vi "adam-ALL-IOs-panel.vi"(0 "VISA Refnum in":refnum<visa-resource-name>, 1 "ADAM-5000-data-current":T3, 3 "Digital Outputs":T4, 4 "Analog Outputs":T6, 5 "error in (no error)":errorcluster, 6 "Module Type":T10(ring), 7 "chassis-slot":i32=5, 9 "cmd-response in":T1, 10 "Chassis Settings":T8, 11 "reference":refnum<vi>) -> (12 "slot: x":T9, 14 "VISA Refnum out":refnum<visa-resource-name>, 15 "ADAM-5000-data-new":T3, 18 "cmd-response out":T1, 19 "error out":errorcluster)   [LabVIEW 2020]
uses:
  controls/digital-output-cluster.ctl
  controls/digitial-input-cluster.ctl
  controls/analog-input-cluster.ctl
  controls/thermocouple-input-cluster.ctl
  controls/adam-module-select-tab.ctl
  controls/adam-5000-serial-settings.ctl
  controls/analog-output-cluster.ctl
  controls/adam-5000-all-module-datas.ctl
  controls/adam-5000-cmd-response.ctl
panel:
  out "Analog Inputs":T2
  out "Digital Inputs":T5
  out "Thermocouple Inputs (degC)":T7
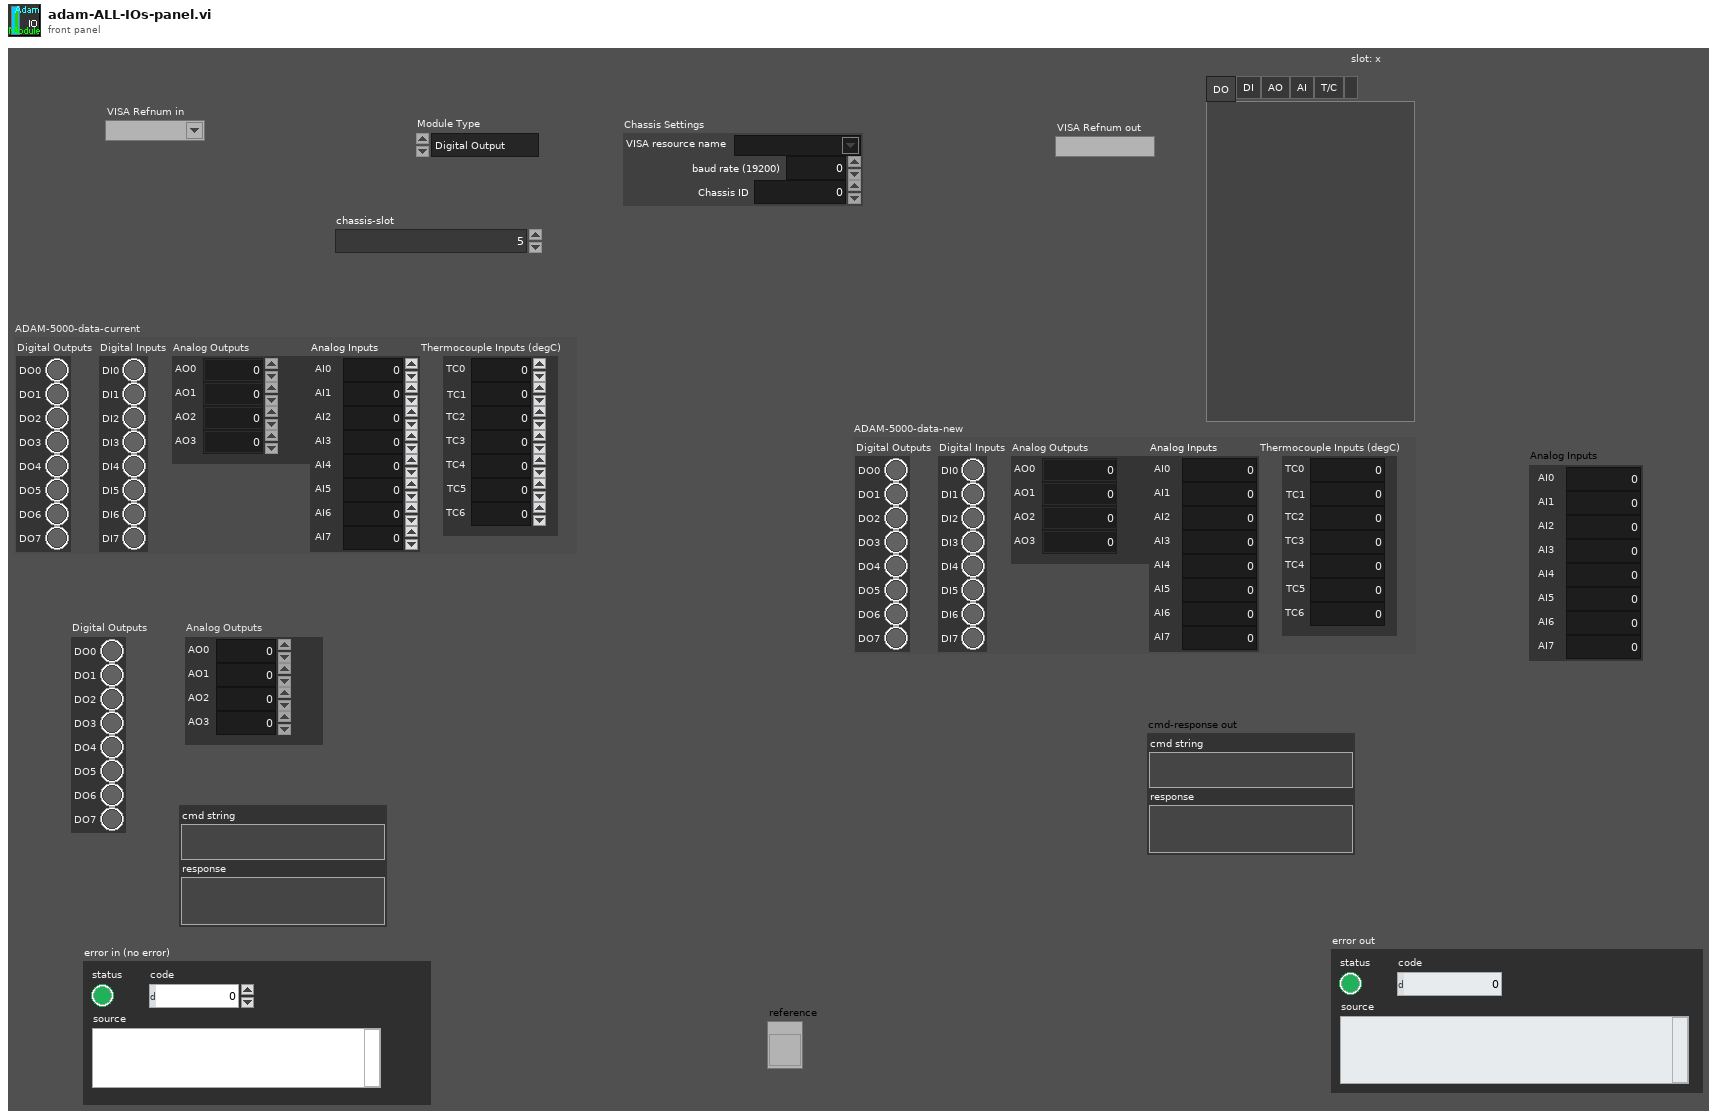
[diagram p1: front panel]
types:
  T1 = typedef "adam-5000-cmd-response.ctl" = cluster{"cmd string":string, "response":string}
  T2 = typedef "analog-input-cluster.ctl" = cluster{"AI0":dbl, "AI1":dbl, "AI2":dbl, "AI3":dbl, "AI4":dbl, "AI5":dbl, "AI6":dbl, "AI7":dbl}
  T3 = typedef "adam-5000-all-module-datas.ctl" = cluster{"Digital Outputs":T4, "Digital Inputs":T5, "Analog Outputs":T6, "Analog Inputs":T2, "Thermocouple Inputs (degC)":T7}
  T4 = typedef "digital-output-cluster.ctl" = cluster{"DO0":bool, "DO1":bool, "DO2":bool, "DO3":bool, "DO4":bool, "DO5":bool, "DO6":bool, "DO7":bool}
  T5 = typedef "digitial-input-cluster.ctl" = cluster{"DI0":bool, "DI1":bool, "DI2":bool, "DI3":bool, "DI4":bool, "DI5":bool, "DI6":bool, "DI7":bool}
  T6 = typedef "analog-output-cluster.ctl" = cluster{"AO0":dbl, "AO1":dbl, "AO2":dbl, "AO3":dbl}
  T7 = typedef "thermocouple-input-cluster.ctl" = cluster{"TC0":dbl, "TC1":dbl, "TC2":dbl, "TC3":dbl, "TC4":dbl, "TC5":dbl, "TC6":dbl}
  T8 = typedef "adam-5000-serial-settings.ctl" = cluster{"VISA resource name":refnum<visa-resource-name>, "baud rate (19200)":u32, "Chassis ID":u8}
  T9 = typedef "adam-module-select-tab.ctl" = enum32{"DO", "DI", "AO", "AI", "T/C", ""}
  T10 = enum16{"Digital Output", "Digital Input", "Analog Output", "Analog Input", "Thermocouple", "Power Relay", "empty"}
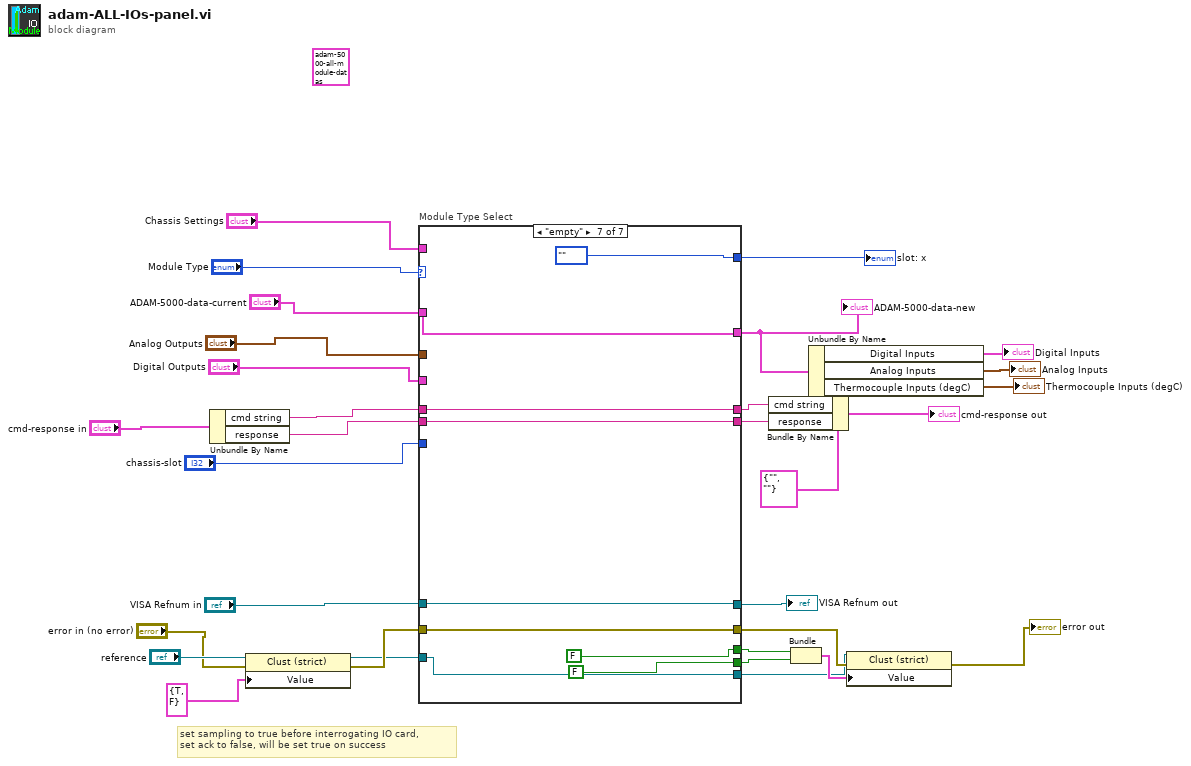
[diagram p0: block diagram]
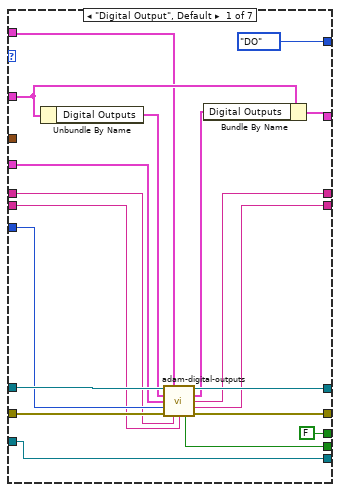
[diagram p2: hidden frame]
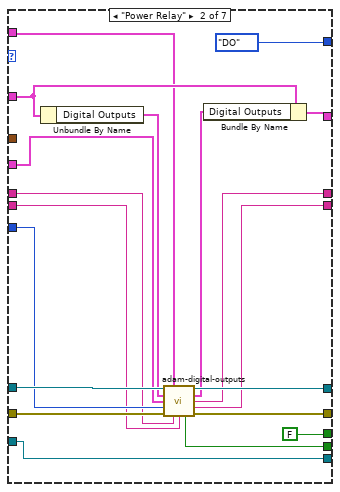
[diagram p3: hidden frame]
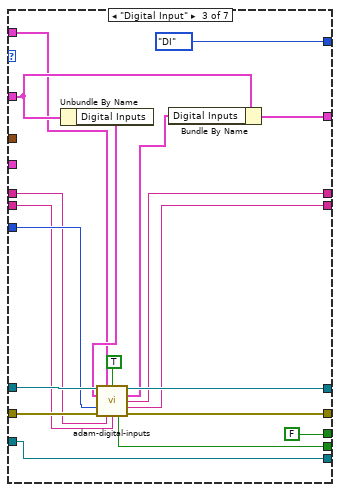
[diagram p4: hidden frame]
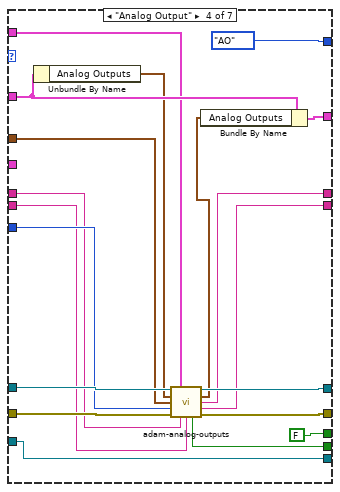
[diagram p5: hidden frame]
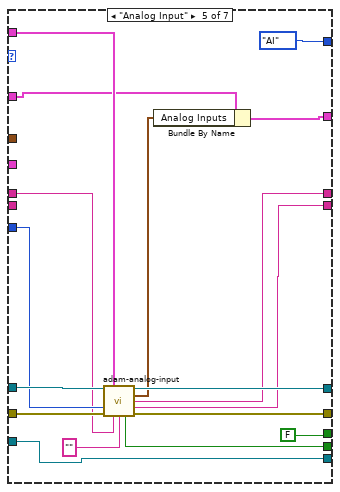
[diagram p6: hidden frame]
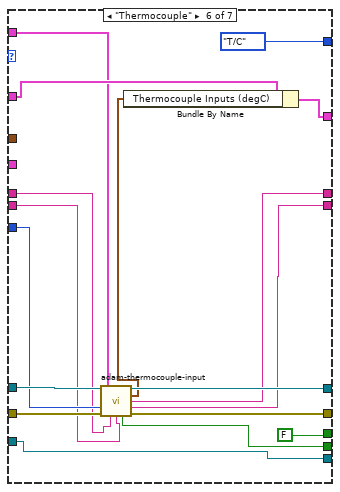
[diagram p7: hidden frame]
diagram:
  (unwired) T3 {"Digital Outputs"={"DO0"=FALSE, "DO1"=FALSE, "DO2"=FALSE, "DO3"=FALSE, "DO4"=FALSE, "DO5"=FALSE, "DO6"=FALSE, "DO7"=FALSE}, "Digital Inputs"={"DI0"=FALSE, "DI1"=FALSE, "DI2"=FALSE, "DI3"=FALSE, "DI4"=FALSE, "DI5"=FALSE, "DI6"=FALSE, "DI7"=FALSE}, "Analog Outputs"={"AO0"=0.0, "AO1"=0.0, "AO2"=0.0, "AO3"=0.0}, "Analog Inputs"={"AI0"=0.0, "AI1"=0.0, "AI2"=0.0, "AI3"=0.0, "AI4"=0.0, "AI5"=0.0, "AI6"=0.0, "AI7"=0.0}, "Thermocouple Inputs (degC)"={"TC0"=0.0, "TC1"=0.0, "TC2"=0.0, "TC3"=0.0, "TC4"=0.0, "TC5"=0.0, "TC6"=0.0}} ("ADAM-5000-data-typedefs")
  # "set sampling to true before interrogating IO card,\nset ack to false, will be set true on success"
  n1 = Unbundle By Name("cmd-response in") -> ("cmd string"=w19:string, "response"=w20:string)
  n2 = property on="Property Node" class="Clust (strict)"(reference="reference", error in="error in (no error)", "Value"=cluster{"Sampling":bool, "Ack":bool} {"Sampling"=TRUE, "Ack"=FALSE}) -> (reference out=w7:refnum<vi>, error out=w9:errorcluster)
  n3 = case "Module Type Select" shown="\"empty\"" "Module Type" {
    tunnel: "ADAM-5000-data-current" -> [w48 w67 w82 w106 w117 w141 w143]
    tunnel: [adam-module-select-tab."DO" ("slot: 0") adam-module-select-tab."DO" ("slot: 0") adam-module-select-tab."DI" ("slot: 0") adam-module-select-tab."AO" ("slot: 0") adam-module-select-tab."AI" ("slot: 0") adam-module-select-tab."T/C" ("slot: 0") adam-module-select-tab."" ("slot: 0")] -> w26
    tunnel: [w49 w68 w87 w105 w116 w140 w143] -> w24
    tunnel: "Chassis Settings" -> [w38 w57 w75 w97 w124 w134 _]
    tunnel: "chassis-slot" -> [w41 w60 w80 w98 w119 w133 _]
    tunnel: "VISA Refnum in" -> [w47 w66 w86 w102 w123 w138 w144]
    tunnel: w9 -> [w46 w65 w85 w104 w122 w137 w145]
    tunnel: [w45 w64 w84 w103 w121 w136 w145] -> w6
    tunnel: [w44 w63 w83 w101 w120 w135 w144] -> w28
    tunnel: [w39 w58 w76 w95 w118 w129 w147] -> w13
    tunnel: w20 -> [w36 w55 w78 w94 _ w131 w147]
    tunnel: w19 -> [w37 w56 w79 w93 w113 w132 w148]
    tunnel: [w34 w52 w71 w90 w109 w126 FALSE ("Sampling")] -> w17
    tunnel: [w40 w59 w77 w96 w114 w130 w148] -> w14
    tunnel: [FALSE ("cmd aknowledged") FALSE ("Sampling") FALSE ("Sampling") FALSE ("Sampling") FALSE ("Sampling") FALSE ("Sampling") FALSE ("cmd aknowledged")] -> w18
    tunnel: "Digital Outputs" -> [w35 w54 _ _ _ _ _]
    tunnel: "Analog Outputs" -> [_ _ _ w92 _ _ _]
    tunnel: w7 -> [w32 w51 w70 w89 w108 w125 w142]
    tunnel: [w32 w51 w70 w89 w108 w125 w142] -> w3
    frame "Digital Output", Default {
      n4 = Unbundle By Name(w48) -> ("Digital Outputs"=w43:T4)
      n5 = call "adam-digital-outputs.vi"("VISA Refnum in"=w47, "Chassis Settings"=w38, "Current DO State"=w43, "DO Control"=w35, "chassis-slot"=w41, "error in (no error)"=w46, "cmd-in"=w37, "ack char"=w36) -> ("VISA Refnum out"=w44:refnum<visa-resource-name>, "New DO State"=w42:T4, "cmd-out"=w40:string, "acknowledge char"=w39:string, "cmd aknowledged"=w34:bool, "error out"=w45:errorcluster)  [unwired: 2 in]
      n6 = Bundle By Name(cluster=w48, "Digital Outputs"=w42) -> (w49:T3)
    }
    frame "Power Relay" {
      n7 = Unbundle By Name(w67) -> ("Digital Outputs"=w62:T4)
      n8 = call "adam-digital-outputs.vi"("VISA Refnum in"=w66, "Chassis Settings"=w57, "Current DO State"=w62, "DO Control"=w54, "chassis-slot"=w60, "error in (no error)"=w65, "cmd-in"=w56, "ack char"=w55) -> ("VISA Refnum out"=w63:refnum<visa-resource-name>, "New DO State"=w61:T4, "cmd-out"=w59:string, "acknowledge char"=w58:string, "cmd aknowledged"=w52:bool, "error out"=w64:errorcluster)  [unwired: 2 in]
      n9 = Bundle By Name(cluster=w67, "Digital Outputs"=w61) -> (w68:T3)
    }
    frame "Digital Input" {
      n10 = Unbundle By Name(w82) -> ("Digital Inputs"=w81:T5)
      n11 = call "adam-digital-inputs.vi"("VISA Refnum in"=w86, "Chassis Settings"=w75, "sample?"=TRUE, "Current DI State"=w81, "chassis-slot"=w80, "error in (no error)"=w85, "cmd-in"=w79, "ack char"=w78) -> ("VISA Refnum out"=w83:refnum<visa-resource-name>, "New DI State"=w73:T5, "cmd-out"=w77:string, "acknowledge char"=w76:string, "cmd aknowledged"=w71:bool, "error out"=w84:errorcluster)  [unwired: 2 in]
      n12 = Bundle By Name(cluster=w82, "Digital Inputs"=w73) -> (w87:T3)
    }
    frame "Analog Output" {
      n13 = Unbundle By Name(w106) -> ("Analog Outputs"=w100:T6)
      n14 = call "adam-analog-outputs.vi"("VISA Refnum in"=w102, "Chassis Settings"=w97, "Current AO States"=w100, "Analog Outputs in"=w92, "chassis-slot"=w98, "error in (no error)"=w104, "Last cmd"=w93, "last ack message"=w94) -> ("VISA Refnum out"=w101:refnum<visa-resource-name>, "Analog Outputs out"=w99:T6, "cmd output"=w96:string, "ack message"=w95:string, "cmd aknowledged"=w90:bool, "error out"=w103:errorcluster)  [unwired: 2 in]
      n15 = Bundle By Name(cluster=w106, "Analog Outputs"=w99) -> (w105:T3)
    }
    frame "Analog Input" {
      n16 = call "adam-analog-input.vi"("VISA Refnum in"=w123, "Chassis Settings"=w124, "chassis-slot"=w119, "error in (no error)"=w122, "last cmd in"=w113, "last read buffer"="") -> ("VISA Refnum out"=w120:refnum<visa-resource-name>, "Analog Inputs"=w112:T2, "cmd out"=w114:string, "read-buffer out"=w118:string, "cmd aknowledged"=w109:bool, "error out"=w121:errorcluster)  [unwired: 4 in]
      n17 = Bundle By Name(cluster=w117, "Analog Inputs"=w112) -> (w116:T3)
    }
    frame "Thermocouple" {
      n18 = call "adam-thermocouple-input.vi"("VISA Refnum in"=w138, "Chassis Settings"=w134, "chassis-slot"=w133, "error in (no error)"=w137, "last cmd in"=w132, "last read buffer"=w131) -> ("VISA Refnum out"=w135:refnum<visa-resource-name>, "Thermocouple Inputs (degC)"=w128:T7, "cmd out"=w130:string, "read-buffer out"=w129:string, "cmd aknowledged"=w126:bool, "error out"=w136:errorcluster)  [unwired: 4 in]
      n19 = Bundle By Name(cluster=w141, "Thermocouple Inputs (degC)"=w128) -> (w140:T3)
    }
    frame "empty" {
    }
  }
  "slot: x" <- w26
  "VISA Refnum out" <- w28
  "ADAM-5000-data-new" <- w24
  n20 = Bundle By Name(cluster=T1 {"cmd string"="", "response"=""} ("cmd-response:0"), "cmd string"=w14, "response"=w13) -> (→"cmd-response out":T1)
  n21 = Bundle("cmd aknowledged"=w18, "Sampling"=w17) -> (w4:cluster{"cmd aknowledged":bool, "Sampling":bool})  [unwired: 1 in]
  n22 = Unbundle By Name(w24) -> ("Digital Inputs"=→"Digital Inputs":T5, "Analog Inputs"=→"Analog Inputs":T2, "Thermocouple Inputs (degC)"=→"Thermocouple Inputs (degC)":T7)
  n23 = property on="Property Node" class="Clust (strict)"(reference=w3, error in=w6, "Value"=w4) -> (error out=→"error out":errorcluster)  [unwired: 1 out]
